vi "Amplifier Daemon Test Interface.vi"() -> ()   [LabVIEW 2012, in "MultiClamp 700B Controls.lvlib"]
uses:
  MultiClamp 700B Controls.lvlib
panel:
  in  "Error in":errorcluster
  in  "Capacitance Compensation":T1
  in  "Capacitance Compensation":cluster{"Iterations":i32, "Timeout [ms]":u32}
  in  "Target Amplitude":dbl
  in  "Autotune":bool
  out "Test Signal":waveform(dbl)(graph)
  in  "Holding Potential":T2 {"Holding Potential [mV]" scale=-100.0..100.0}
  in  "Reset":bool
  in  "Exit":bool
  out "Error Out":errorcluster
  in  "Channel":u16(ring) items=["Channel 1", "Channel 2"]
  in  "pszSerialNum":string="00106392"
  in  "Gain":u16(ring) items=["1"=1, "2"=2, "5"=5, "10"=10, "20"=20, "50"=50, "100"=100, "200"=200, "500"=500, "1000"=1000, "2000"=2000]
  in  "Test Signal Parameters and Offset":T3 {"Frequency\n[hz]" items=["2 hz "=2, "5 hz"=5, "10 hz "=10, "20 hz"=20, "50 hz"=50, "60 hz"=60, "100 hz"=100, "200 hz"=200, "500 hz"=500, "1000 hz"=1000]}
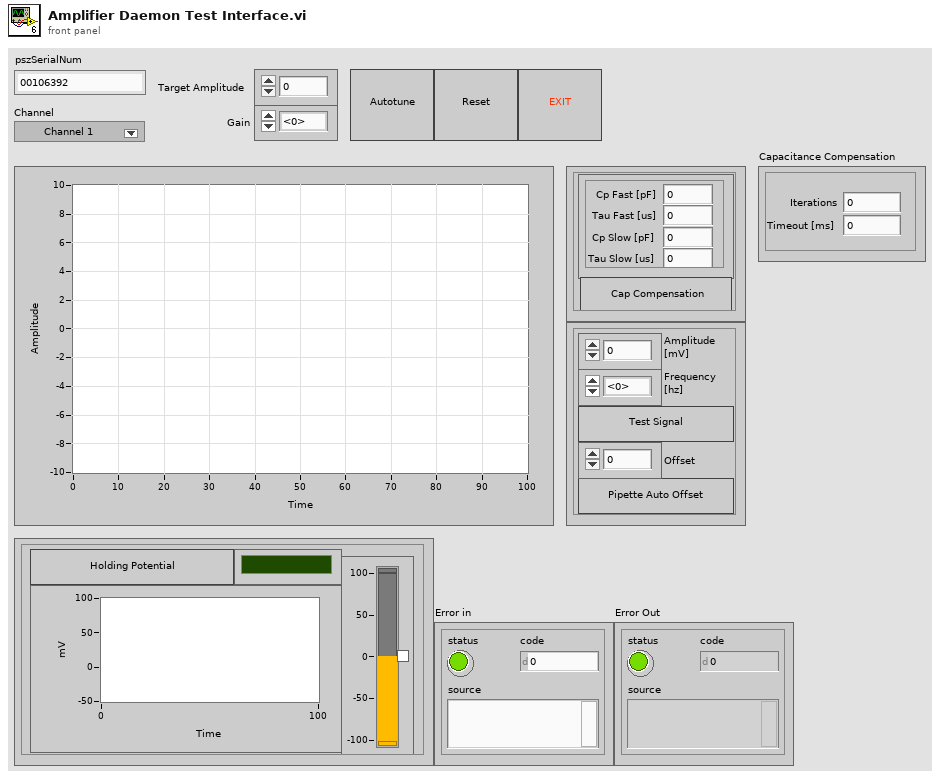
[diagram p1: front panel]
types:
  T1 = cluster{"Capacitance Compensation Indicators":cluster{"Cp Fast [pF]":dbl, "Tau Fast [us]":dbl, "Cp Slow [pF]":dbl, "Tau Slow [us]":dbl}, "Capacitance Compensation 2":bool}
  T2 = cluster{"Holding Potential Chart":dbl, "Holding Potential":bool, "Holding Potential [mV]":i32, "Indicator 17":cluster{"Holding Potential Led":bool}}
  T3 = cluster{"Pipette Offset":bool, "Test Signal":bool, "Amplitude\n[mV]":i32, "Frequency\n[hz]":u16, "Offset":dbl}
  T4 = cluster{"Timeout [ms]":refnum<vi>, "Iterations":refnum<vi>, "Compensate":refnum<vi>, "Capacitance Compensation Indicators":refnum<vi>}
  T5 = cluster{"Autotune Gain":refnum<vi>, "Target Amplitude [mV]":refnum<vi>}
  T6 = cluster{"Test Signal":refnum<vi>, "Amplitude [mV]":refnum<vi>, "Frequency [hz]":refnum<vi>}
  T7 = cluster{"Pipette Offset":refnum<vi>, "Offset Value [mV]":refnum<vi>}
  T8 = cluster{"Holding Potential [mV]":refnum<vi>, "Holding Potential":refnum<vi>, "Holding Potential Indicator":refnum<vi>}
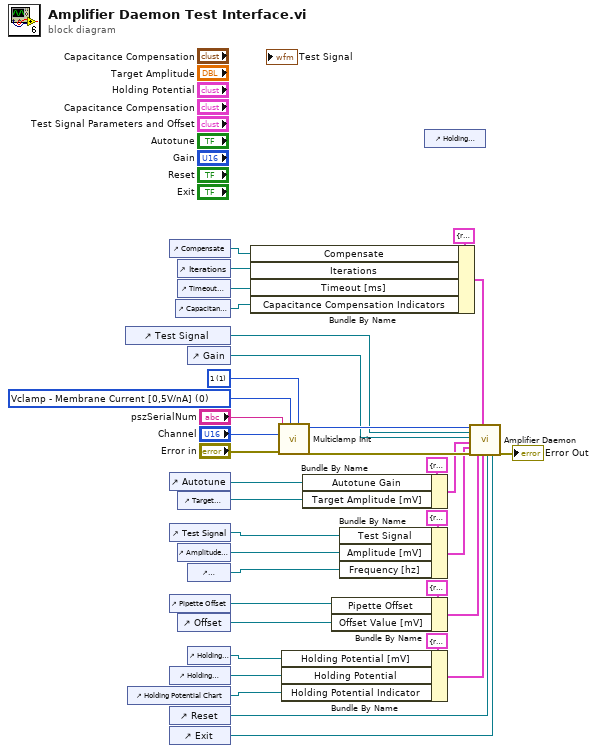
[diagram p0: block diagram]
diagram:
  w33 = u16 1 items=["1"=1, "2"=2, "5"=5, "10"=10, "20"=20, "50"=50, "100"=100, "200"=200, "500"=500, "1000"=1000, "2000"=2000] ("Gain")
  w34 = u16 0 items=["Vclamp - Membrane Current [0,5V/nA]", "Vclamp - Membrane Potential [10mV/10mV]", "Vclamp - Pipette Potential [1mV/mV]", "Vclamp - 100x AC Membrane Potential  [100mV/mV]", "Vclamp - External Command Potential  [50mV/mV]", "Vclamp - Auxiliary 1 Potential  [10mV/mV]", "Vclamp - Auxiliary 2 Current  [0,01V/nA]", "Iclamp - Membrane Potential  [10mV/mV]", "Iclamp - Membran Current  [0,5V/nA]", "Iclamp - Command Current  [0,5V/nA]", "Iclamp - 100x AC Membrane Potential  [100mV/mV]", "Iclamp - External Command Current [2,5V/nA]", "Iclamp - Auxiliary 1 Potential   [10mV/mV]", "Iclamp - Auxiliary 2 Current   [0,01V/nA]"] ("Primary Output")
  n1 = control-ref of="Test Signal"() -> (w21:refnum<vi>)
  n2 = control-ref of="Holding Potential Chart"() -> (w23:refnum<vi>)
  n3 = control-ref of="Compensate"() -> (w4:refnum<vi>)
  n4 = control-ref of="Autotune"() -> (w11:refnum<vi>)
  n5 = control-ref of="Test Signal"() -> (w15:refnum<vi>)
  n6 = control-ref of="Pipette Offset"() -> (w18:refnum<vi>)
  n7 = control-ref of="Holding Potential"() -> (w24:refnum<vi>)
  n8 = control-ref of="Reset"() -> (w28:refnum<vi>)
  n9 = control-ref of="Exit"() -> (w29:refnum<vi>)
  n10 = control-ref of="Capacitance Compensation Indicators"() -> (w3:refnum<vi>)
  n11 = control-ref of="Iterations"() -> (w7:refnum<vi>)
  n12 = control-ref of="Timeout [ms]"() -> (w6:refnum<vi>)
  n13 = control-ref of="Target Amplitude"() -> (w8:refnum<vi>)
  n14 = control-ref of="Amplitude [mV]"() -> (w14:refnum<vi>)
  n15 = control-ref of="Offset"() -> (w17:refnum<vi>)
  n16 = control-ref of="Gain"() -> (w22:refnum<vi>)
  n17 = control-ref of="Frequency [hz]"() -> (w13:refnum<vi>)
  n18 = control-ref of="Holding Potential [mV]"() -> (w26:refnum<vi>)
  n19 = Bundle By Name(cluster=T4 {"Timeout [ms]"=refnum, "Iterations"=refnum, "Compensate"=refnum, "Capacitance Compensation Indicators"=refnum} ("Capacitance Compensation"), "Compensate"=w4, "Iterations"=w7, "Timeout [ms]"=w6, "Capacitance Compensation Indicators"=w3) -> (w2:T4)
  n20 = call "Multiclamp Init.vi"("Gain"=w33, "Primary Output"=w34, "error in (no error)"="Error in", "Channel"="Channel", "pszSerialNum"="pszSerialNum") -> ("error out"=w31:errorcluster, "Handler"=w32:i32)  [unwired: 4 in, 1 out]
  n21 = Bundle By Name(cluster=T8 {"Holding Potential [mV]"=refnum, "Holding Potential"=refnum, "Holding Potential Indicator"=refnum} ("Holding Potential"), "Holding Potential [mV]"=w26, "Holding Potential"=w24, "Holding Potential Indicator"=w23) -> (w25:T8)
  n22 = Bundle By Name(cluster=T5 {"Autotune Gain"=refnum, "Target Amplitude [mV]"=refnum} ("Autotune Gain"), "Autotune Gain"=w11, "Target Amplitude [mV]"=w8) -> (w9:T5)
  n23 = Bundle By Name(cluster=T7 {"Pipette Offset"=refnum, "Offset Value [mV]"=refnum} ("Pipette Offset"), "Pipette Offset"=w18, "Offset Value [mV]"=w17) -> (w19:T7)
  n24 = Bundle By Name(cluster=T6 {"Test Signal"=refnum, "Amplitude [mV]"=refnum, "Frequency [hz]"=refnum} ("Test Signal"), "Test Signal"=w15, "Amplitude [mV]"=w14, "Frequency [hz]"=w13) -> (w12:T6)
  n25 = control-ref of="Holding Potential Led"() -> ()  [unwired: 1 out]
  n26 = call "Amplifier Daemon.vi"("Multiclamp Reference"=w32, "Signal"=w21, "Gain"=w22, "Autotune Gain"=w9, "Test Signal"=w12, "Error In"=w31, "Capacitance Compensation"=w2, "Pipette Offset"=w19, "Holding Potential"=w25, "Reset"=w28, "Exit"=w29) -> ("Error Out"=→"Error Out":errorcluster)  [unwired: 8 in]
